vi "Read Levels.vi"(8 "error in (no error)":errorcluster, 11 "VoiceMeeterRemote in":refnum<class "VoiceMeeterRemote.lvclass">) -> (0 "error out":errorcluster, 2 "Levels":T1, 3 "VoiceMeeterRemote out":refnum<class "VoiceMeeterRemote.lvclass">)   [LabVIEW 2020, in "VoiceMeeterRemote.lvlib" / "VoiceMeeterRemote.lvclass"]
doc: "Reads all audio levels for all channels for all input and outputs in Voicemeeter. Each cluster entry is grouped by input or output index and contains a cluster with a value array with each element corresponding to each channel available for that input or output. For instance, A1 has 2 channels but B1 has 8 channels.\n\n<b>Pre Fader</b> is the raw value ignoring any processing.\n<b>Post Fader</b> is the audio level after gain adjustment is applied regardless of the channel's mute state.\n<b>Post Mute</b> is the same as Post Fader but will be at minimum when the channel is muted.\n<b>Output</b>"
uses:
  VoiceMeeterRemote.lvclass
  Levels.ctl
  Device Channels.ctl
  VoiceMeeterRemote.lvclass/VoiceMeeterRemote.ctl
  VoiceMeeterRemote.lvlib
panel:
  out "Array":i32[][](array[numeric])
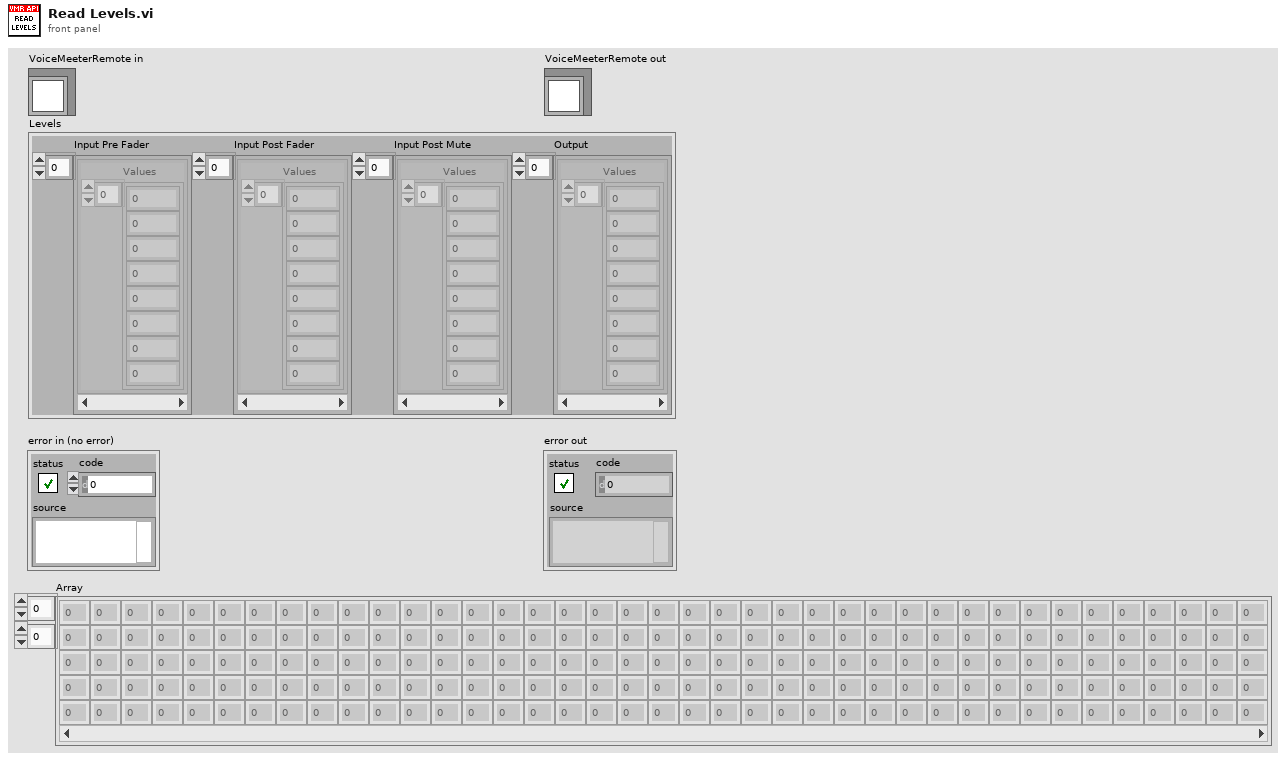
[diagram p1: front panel]
types:
  T1 = typedef "VoiceMeeterRemote.lvlib/Levels.ctl" = cluster{"Input Pre Fader":T2[], "Input Post Fader":T2[], "Input Post Mute":T2[], "Output":T2[]}
  T2 = typedef "VoiceMeeterRemote.lvlib/Device Channels.ctl" = cluster{"Values":sgl[]}
  T3 = typedef "VoiceMeeterRemote.lvlib/Voicemeeter Type.ctl" = enum16{"Unknown", "Voicemeeter", "Banana", "Potato", "Potato x64"}
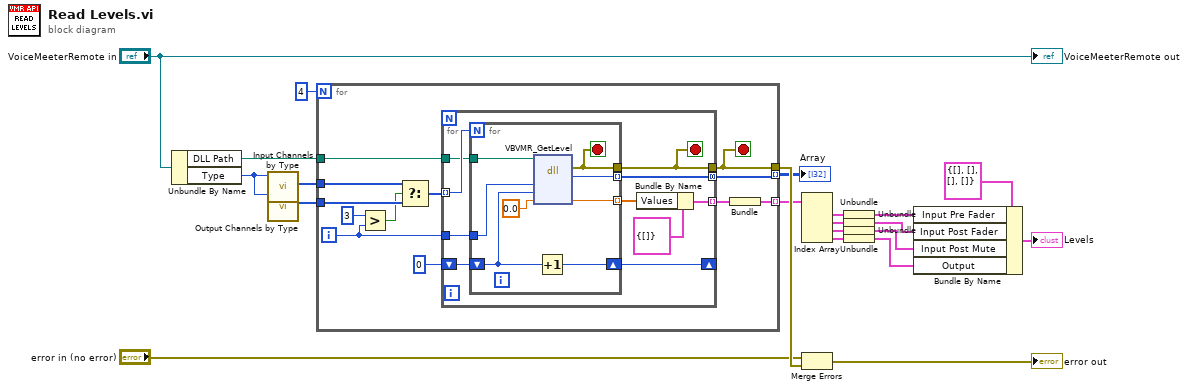
[diagram p0: block diagram]
diagram:
  n1 = Unbundle By Name("VoiceMeeterRemote in") -> ("DLL Path"=w17:path, "Type"=w2:T3)
  n2 = call "Input Channels by Type.vi"("Voicemeeter Type"=w2) -> ("Channel Count"=w18:i32[])  [unwired: 10 in]
  n3 = call "Output Channels by Type.vi"("Voicemeeter Type"=w2) -> ("Channel Count"=w1:i32[])  [unwired: 10 in]
  n4 = for {
    N: 4 -> [_]
    tunnel: w18 -> [w27]
    tunnel: w17 -> [w33]
    tunnel: [w30] -> w15 mode=indexing
    tunnel: [w31] -> w21
    tunnel: [w28] -> w3 mode=indexing
    tunnel: w1 -> [w26]
    i -> [w25]
    stop <- w31 stop-if-true
    n5 = Greater?(x=3, y=w25) -> (0:w23:bool)
    n6 = Select(t=w27, s=w23, f=w26) -> (s? t:f=w22:i32[])
    n7 = for {
      tunnel: w22 -> [w43] mode=indexing
      tunnel: w33 -> [w42]
      shift-right: [w40] -> _
      shift-left: 0 -> [w41]
      tunnel: w25 -> [w39]
      tunnel: [w36] -> w29 mode=indexing
      tunnel: [w35] -> w31
      tunnel: [w34] -> w28 mode=concatenating
      stop <- w35 stop-if-true
      n8 = for {
        N: w43 -> [_]
        tunnel: w42 -> [w50]
        shift-right: [w51] -> w40
        shift-left: w41 -> [w48]
        tunnel: w39 -> [w49]
        tunnel: [w46] -> w35
        tunnel: [w45] -> w37 mode=indexing
        tunnel: [w44] -> w34 mode=indexing
        stop <- w46 stop-if-true
        n9 = dll-call lib="C:/Program Files/National Instruments/LabVIEW 2022/user.lib/VoicemeeterRemote64/VoicemeeterRemote64.*" fn="VBVMR_GetLevel"(path in=w50, "nType"=w49, "nuChannel"=w48, "pValue"=sgl 0.0) -> (error out=w46:errorcluster, "return type"=w44:i32, "pValue"=w45:sgl)  [unwired: 4 in, 1 out]
        n10 = Increment(x=w48) -> (x+1=w51:i32)
      }
      n11 = Bundle By Name(cluster=T2 {"Values"=[]} ("Device Channels"), "Values"=w37) -> (w36:T2)
    }
    n12 = Bundle(w29) -> (w30:cluster{T2[]})  [unwired: 1 in]
  }
  "Array" <- w3
  n13 = Index Array(array=w15) -> (element #1=w12:cluster{T2[]}, element #2=w11:cluster{T2[]}, element #3=w9:cluster{T2[]}, element #4=w10:cluster{T2[]})  [unwired: 4 in]
  n14 = Merge Errors("error in (no error)", w21) -> (→"error out":errorcluster)
  n15 = Unbundle(w12) -> (w8:T2[])
  n16 = Unbundle(w11) -> (w7:T2[])
  n17 = Unbundle(w9) -> (w6:T2[])
  n18 = Unbundle(w10) -> (w5:T2[])
  n19 = Bundle By Name(cluster=T1 {"Input Pre Fader"=[], "Input Post Fader"=[], "Input Post Mute"=[], "Output"=[]} ("Levels"), "Input Pre Fader"=w8, "Input Post Fader"=w7, "Input Post Mute"=w6, "Output"=w5) -> (→"Levels":T1)
  "VoiceMeeterRemote out" <- "VoiceMeeterRemote in"
